vi "GetNumVideoDrivers.vi"(8 "No Error":errorcluster) -> (0 "Error Out":errorcluster, 3 "Video Driver Number":i32)   [LabVIEW 2024, in "SDL3.lvlib" / "Video.lvlib"]
doc: "<B>Summary</B>\nGet the number of video drivers compiled into SDL."
uses:
  Video.lvlib
  Lib/SDL3-32.dll
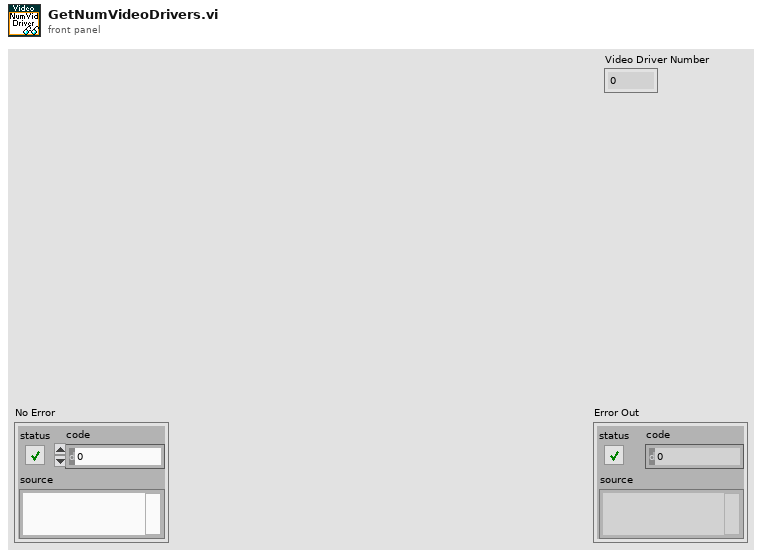
[diagram p1: front panel]
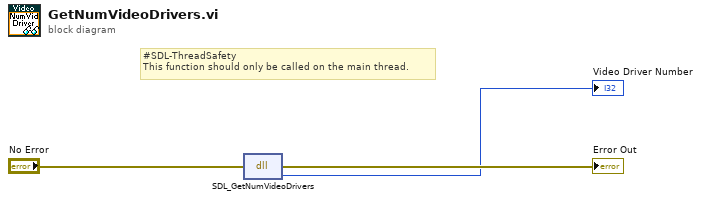
[diagram p0: block diagram]
diagram:
  # "#SDL-ThreadSafety\nThis function should only be called on the main thread."
  n1 = dll-call lib="C:/Users/Thomas/Documents/Projects/LV-SDL3/Lib/SDL3-*.*" fn="SDL_GetNumVideoDrivers"(error in="No Error") -> (error out=→"Error Out":errorcluster, "return type"=→"Video Driver Number":i32)  [unwired: 2 in, 1 out]
